vi "Voltech2.vi"() -> ()   [LabVIEW 2011]
uses:
  <instrlib>/Voltech PM1000+/Public/Configure/Configure Measurements (Normal).vi
  <vilib>/Utility/file.llb/Write To Spreadsheet File (string).vi
  <instrlib>/Voltech PM1000+/Voltech PM1000+.lvlib
panel:
  out "VRMS":dbl[](graph)
  in  "stop":bool
  in  "Normal Measurements":i32[](listbox)=[0, 1, 2, 3, 4, 5, 6]
  out "Current Data Point":i32
  in  "Name of File":string
  out "error out":errorcluster
  in  "VISA resource name 2":refnum<visa-resource-name>
  # "Voltech"
  # "Note to select specific measurements\nHold CTRL and select"
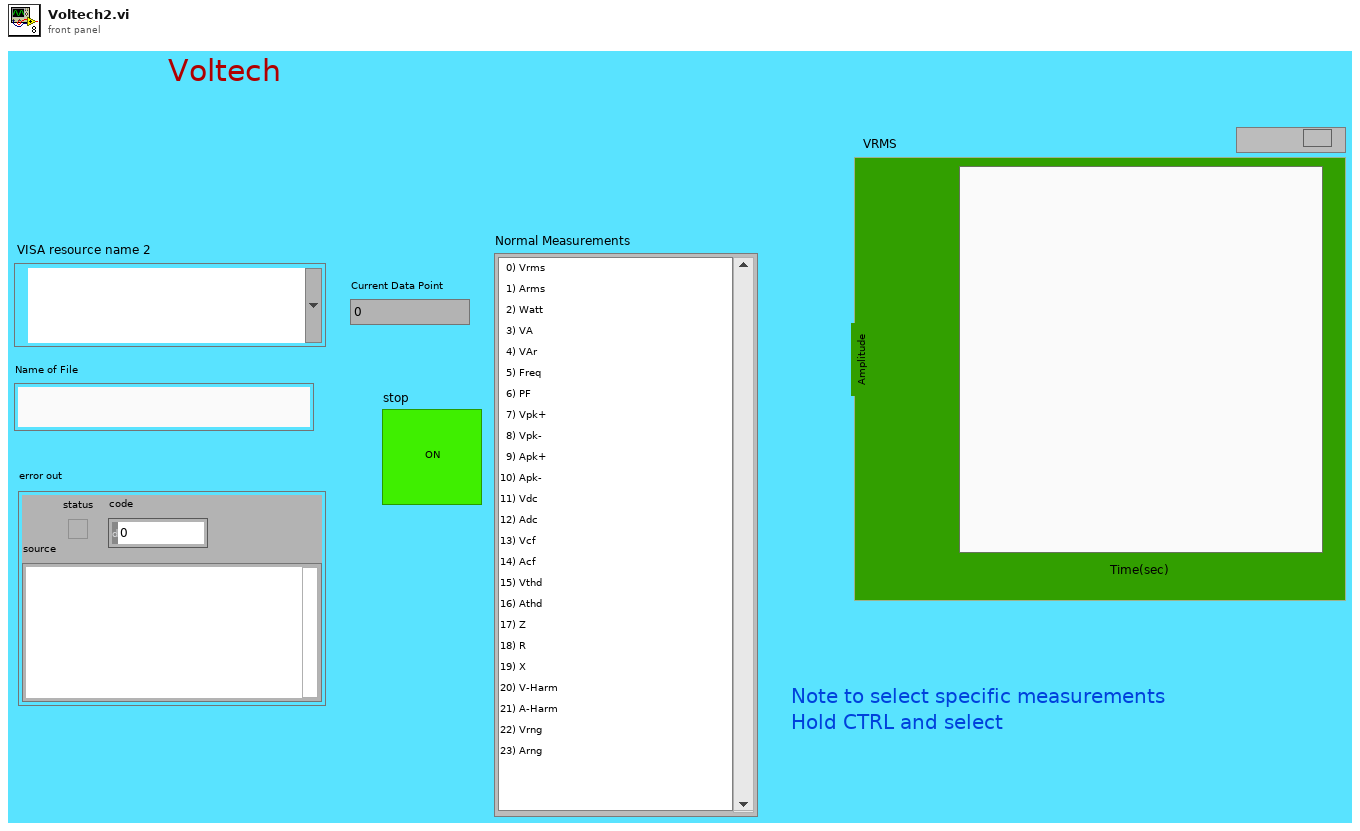
[diagram p1: front panel]
types:
  T1 = enum16{"open", "replace", "create", "open or create", "replace or create", "replace or create with confirmation"}
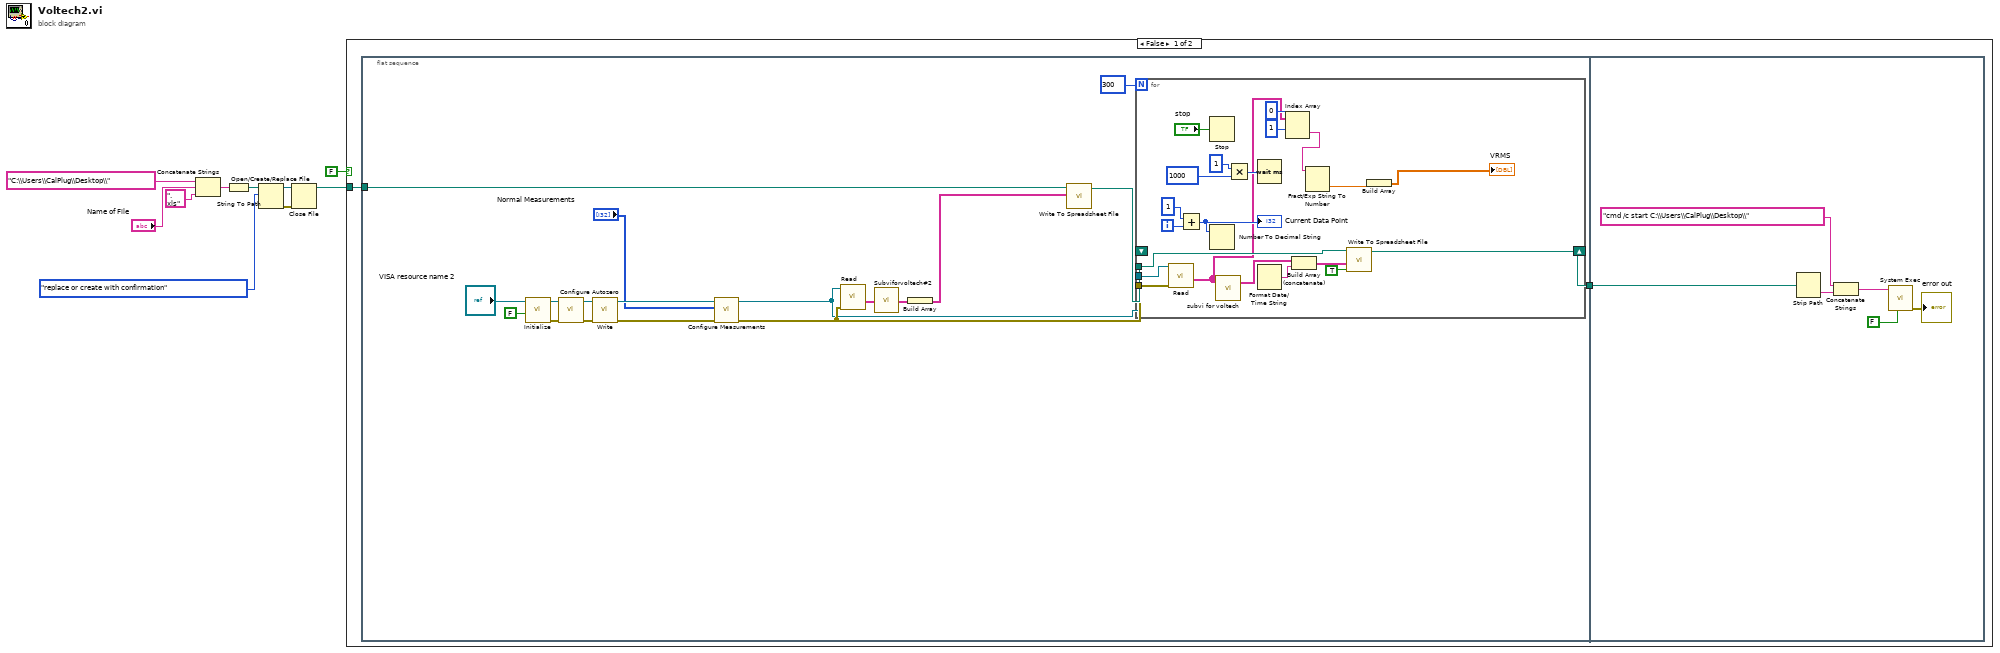
[diagram p0: block diagram]
diagram:
  n1 = Concatenate Strings("C:\\Users\\CalPlug\\Desktop\\" ("string"), "Name of File", ".xls" ("string")) -> (w7:string)
  n2 = String To Path(string=w7) -> (path=w6:path)
  n3 = Open/Create/Replace File(file path (use dialog)=w6, operation (0:open)=T1."replace or create with confirmation") -> (refnum out=w5:refnum<file>, error out=w1:errorcluster)  [unwired: 4 in, 1 out]
  n4 = Close File(refnum=w5, error in=w1) -> (path=w4:path)  [unwired: 1 out]
  n5 = case shown="False" FALSE {
    tunnel: w4 -> [w12 _]
    frame False {
      n6 = flat-sequence {
        tunnel: w12 -> [w19]
        tunnel: [w26] -> w11
        tunnel: w11 -> [w53]
        frame #0 {
          n7 = call <instrlib>:"Initialize.vi"("Reset (True)"=FALSE, "VISA resource name"="VISA resource name 2") -> ("error out"=w28:errorcluster, "VISA resource name out"=w29:refnum<visa-resource-name>)  [unwired: 8 in]
          n8 = call <instrlib>:"Configure Autozero.vi"("error in (no error)"=w28, "VISA resource name"=w29) -> ("error out"=w24:errorcluster, "VISA resource name out"=w25:refnum<visa-resource-name>)  [unwired: 8 in]
          n9 = call <instrlib>:"Write.vi"("error in (no error)"=w24, "VISA resource name"=w25) -> ("error out"=w22:errorcluster, "VISA resource name out"=w23:refnum<visa-resource-name>)  [unwired: 8 in]
          n10 = call-poly <instrlib>:"Configure Measurements.vi"("error in (no error)"=w22, "Normal Measurements"="Normal Measurements", "VISA resource name"=w23) -> ("error out"=w14:errorcluster, "VISA resource name out"=w13:refnum<visa-resource-name>)  [unwired: 7 in]
          n11 = call <instrlib>:"Read.vi"("error in (no error)"=w14, "VISA resource name"=w13) -> ("Measurement Results"=w15:string[][])  [unwired: 7 in, 2 out]
          n12 = call "Subviforvoltech#2.vi"("Measurement Results 2"=w15) -> ("Array"=w21:string[])
          n13 = Build Array(w21) -> (w20:string[][])
          n14 = call-poly <vilib>:"Write To Spreadsheet File.vi"("2D data"=w20, "file path (dialog if empty)"=w19) -> ("new file path (Not A Path if cancelled)"=w18:path)  [unwired: 6 in]
          n15 = for {
            N: 300 ("How many Data Points") -> [_]
            tunnel: w18 -> [w46]
            shift-right: [w44] -> w26
            shift-left: _ -> [_]
            tunnel: w13 -> [w42]
            tunnel: w14 -> [w41]
            i -> [w48]
            n16 = call <instrlib>:"Read.vi"("error in (no error)"=w41, "VISA resource name"=w42) -> ("Measurement Results"=w32:string[][])  [unwired: 7 in, 2 out]
            n17 = Add(x=1, y=w48) -> (x+y=w49:i32)
            "Current Data Point" <- w49
            n18 = Stop(stop? (T)="stop") -> ()
            n19 = Number To Decimal String(number=w49) -> ()  [unwired: 1 in, 1 out]
            n20 = call "subvi for voltech.vi"("Measurement Results 2"=w32) -> ("Array"=w43:string[])  [unwired: 6 in]
            n21 = Multiply(x=u32 1 ("Interval of Data Collection (sec)"), y=u32 1000) -> (x*y=w50:u32)
            n22 = Wait (ms)(milliseconds to wait=w50) -> ()  [unwired: 1 out]
            n23 = Format Date/Time String() -> (date/time string=w38:string)  [unwired: 3 in]
            n24 = Index Array(array=w32, index (row)=1, index (col)=0 ("disabled index (col)")) -> (element=w35:string)
            n25 = Build Array (concatenate)(w43, w38) -> (w39:string[])
            n26 = Fract/Exp String To Number(string=w35) -> (number=w31:dbl)  [unwired: 3 in, 1 out]
            n27 = call-poly <vilib>:"Write To Spreadsheet File.vi"("append to file? (new file:F)"=TRUE, "1D data"=w39, "file path (dialog if empty)"=w46) -> ("new file path (Not A Path if cancelled)"=w44:path)  [unwired: 5 in]
            n28 = Build Array(w31) -> (→"VRMS":dbl[])
          }
        }
        frame #1 {
          n29 = Strip Path(path=w53) -> (name=w52:string)  [unwired: 1 out]
          n30 = Concatenate Strings("cmd /c start C:\\Users\\CalPlug\\Desktop\\" ("string"), w52) -> (w56:string)
          n31 = call <vilib>:"System Exec.vi"("run minimized? (F)"=FALSE, "command line"=w56) -> ("error out"=→"error out":errorcluster)  [unwired: 6 in, 3 out]
        }
      }
    }
    frame True {
    }
  }
